vi "Create Transceiver Thread.vi"(8 "error in (no error)":errorcluster, 9 "Debug Flags":refnum<class "Debug Flags.lvclass">, 10 "Transfer Groups":refnum<class "DSF.Engine.Transfer Group.lvclass">[](array[class]), 11 "Transceiver type":refnum<class "Transceiver.lvclass">) -> (0 "error out":errorcluster, 3 "Transceiver Thread out":refnum<class "Transceiver Thread.lvclass">)   [LabVIEW 2017, in "Data Sharing Framework Engine.lvlib" / "Transceiver Thread.lvclass"]
uses:
  Transceiver Thread.lvclass
  Transceiver/Transceiver.lvclass
  Debug/Debug Flags/Debug Flags.lvclass
  old/dsf core/Source/Engine/Classes/Transfer/DSF.Engine.Transfer Group.lvclass
  Transceiver Thread.lvclass/Transceiver Thread.ctl
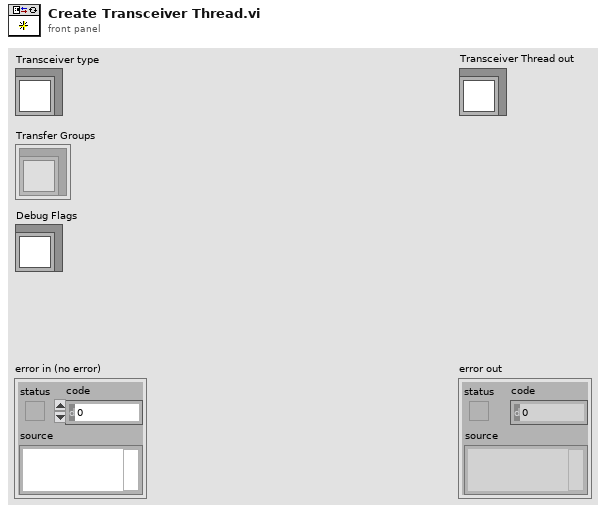
[diagram p1: front panel]
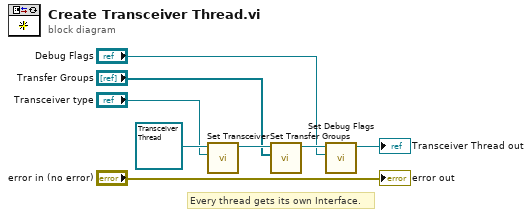
[diagram p0: block diagram]
diagram:
  # "Every thread gets its own Interface."
  n1 = call "Set Transceiver.vi"("Transceiver"="Transceiver type", "Transceiver Thread in"=refnum<class "Transceiver Thread.lvclass"> refnum) -> ("Transceiver Thread out"=w2:refnum<class "Transceiver Thread.lvclass">)  [unwired: 9 in]
  n2 = call "Set Transfer Groups.vi"("Transfer Groups"="Transfer Groups", "Transceiver Thread in"=w2) -> ("Transceiver Thread out"=w6:refnum<class "Transceiver Thread.lvclass">)  [unwired: 9 in]
  n3 = call "Set Debug Flags.vi"("Debug Flags"="Debug Flags", "Transceiver Thread in"=w6) -> ("Transceiver Thread out"=→"Transceiver Thread out":refnum<class "Transceiver Thread.lvclass">)  [unwired: 9 in]
  "error out" <- "error in (no error)"
